vi "SeCrTs-DI Continuous Sequence Check.vi"(9 "output cluster":T1, 10 "DI":bool, 11 "CDT":dbl) -> (1 "Failure case Seq":string, 2 "Boolean Range":bool, 3 "In Range":string)   [LabVIEW 2022 SP3]
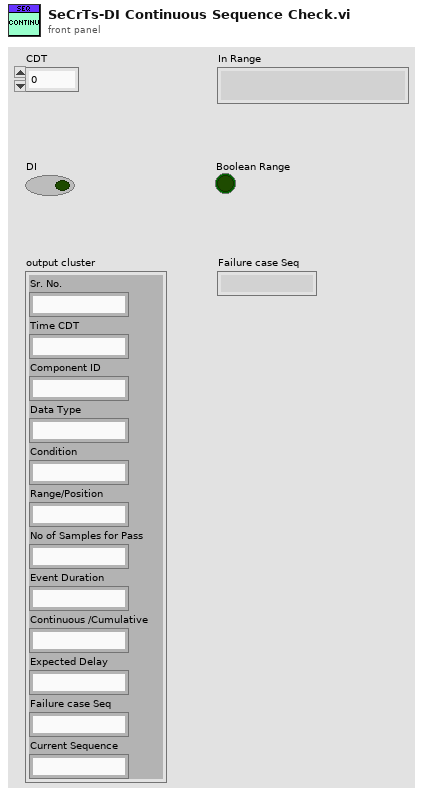
[diagram p1: front panel]
types:
  T1 = cluster{"Sr. No.":string, "Time CDT":string, "Component ID":string, "Data Type":string, "Condition":string, "Range/Position":string, "No of Samples for Pass":string, "Event Duration":string, "Continuous /Cumulative":string, "Expected Delay":string, "Failure case Seq":string, "Current Sequence":string}
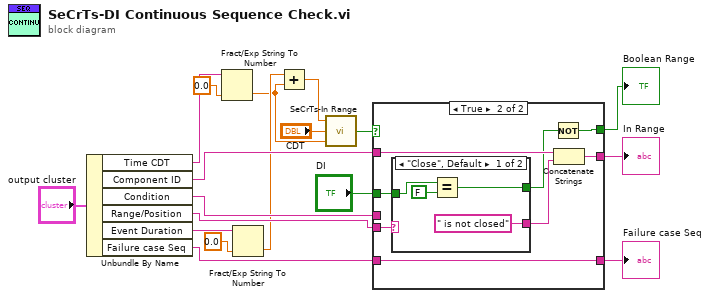
[diagram p0: block diagram]
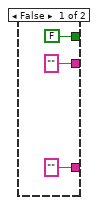
[diagram p2: hidden frame]
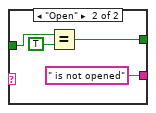
[diagram p3: hidden frame]
diagram:
  n1 = Unbundle By Name("output cluster") -> ("Time CDT"=w9:string, "Component ID"=w11:string, "Condition"=w12:string, "Range/Position"=w13:string, "Event Duration"=w5:string, "Failure case Seq"=w8:string)
  n2 = Fract/Exp String To Number(string=w9, default (0 dbl)=0.0) -> (number=w1:dbl)  [unwired: 2 in, 1 out]
  n3 = Fract/Exp String To Number(string=w5, default (0 dbl)=0.0) -> (number=w2:dbl)  [unwired: 2 in, 1 out]
  n4 = Add(x=w2, y=w1) -> (x+y=w4:dbl)
  n5 = call "SeCrTs-In Range.vi"("Min"=w1, "X"="CDT", "Max"=w4) -> ("In Range"=w7:bool)  [unwired: 2 in]
  n6 = case shown="True" w7 {
    tunnel: w13 -> [_ w24]
    tunnel: w12 -> [_ _]
    tunnel: "DI" -> [_ w23]
    tunnel: w11 -> [_ w29]
    tunnel: ["" w28] -> w18
    tunnel: [FALSE w25] -> w17
    tunnel: w8 -> [_ w27]
    tunnel: ["" ("Failure case Seq") w27] -> w16
    frame False {
    }
    frame True {
      n7 = case shown="\"Close\", Default" w24 {
        tunnel: w23 -> [w32 w37]
        tunnel: [w30 w35] -> w26
        tunnel: [" is not closed" ("string") " is not opened" ("string")] -> w22
        frame "Close", Default {
          n8 = Equal?(x=w32, y=FALSE ("x")) -> (x = y?=w30:bool)
        }
        frame "Open" {
          n9 = Equal?(x=w37, y=TRUE ("x")) -> (x = y?=w35:bool)
        }
      }
      n10 = Not(x=w26) -> (.not. x?=w25:bool)
      n11 = Concatenate Strings(w29, w22) -> (w28:string)
    }
  }
  "In Range" <- w18
  "Boolean Range" <- w17
  "Failure case Seq" <- w16
